vi "ToTable Test.vi"() -> (2 "Pass":bool)   [LabVIEW 2013, in "Table Manager tests.lvlib"]
uses:
  Table Manager tests.lvlib
  <vilib>/NI/Tag Bus/tag/Data Type.ctl
  editor node/Permissions Enum.ctl
  Listbox/Multi Column Listbox.lvclass
  Listbox/Multi Column Listbox.lvclass/Multi Column Listbox.ctl
  Table Manager/Table Manager.lvclass/Table Manager.ctl
  editor node/tag bus configurable plugin editor node.lvclass
  Listbox/Write Listbox.vi
  Table Manager/Write Top VI.vi
  <vilib>/NI/Tag Bus/tag/tag descriptor.lvclass
panel:
  out "error":errorcluster
  in  "Permissions":T1
  in  "data type":T2
  in  "Table":i32(listbox)
  out "error out":errorcluster
  out "table":string[][](array[string])
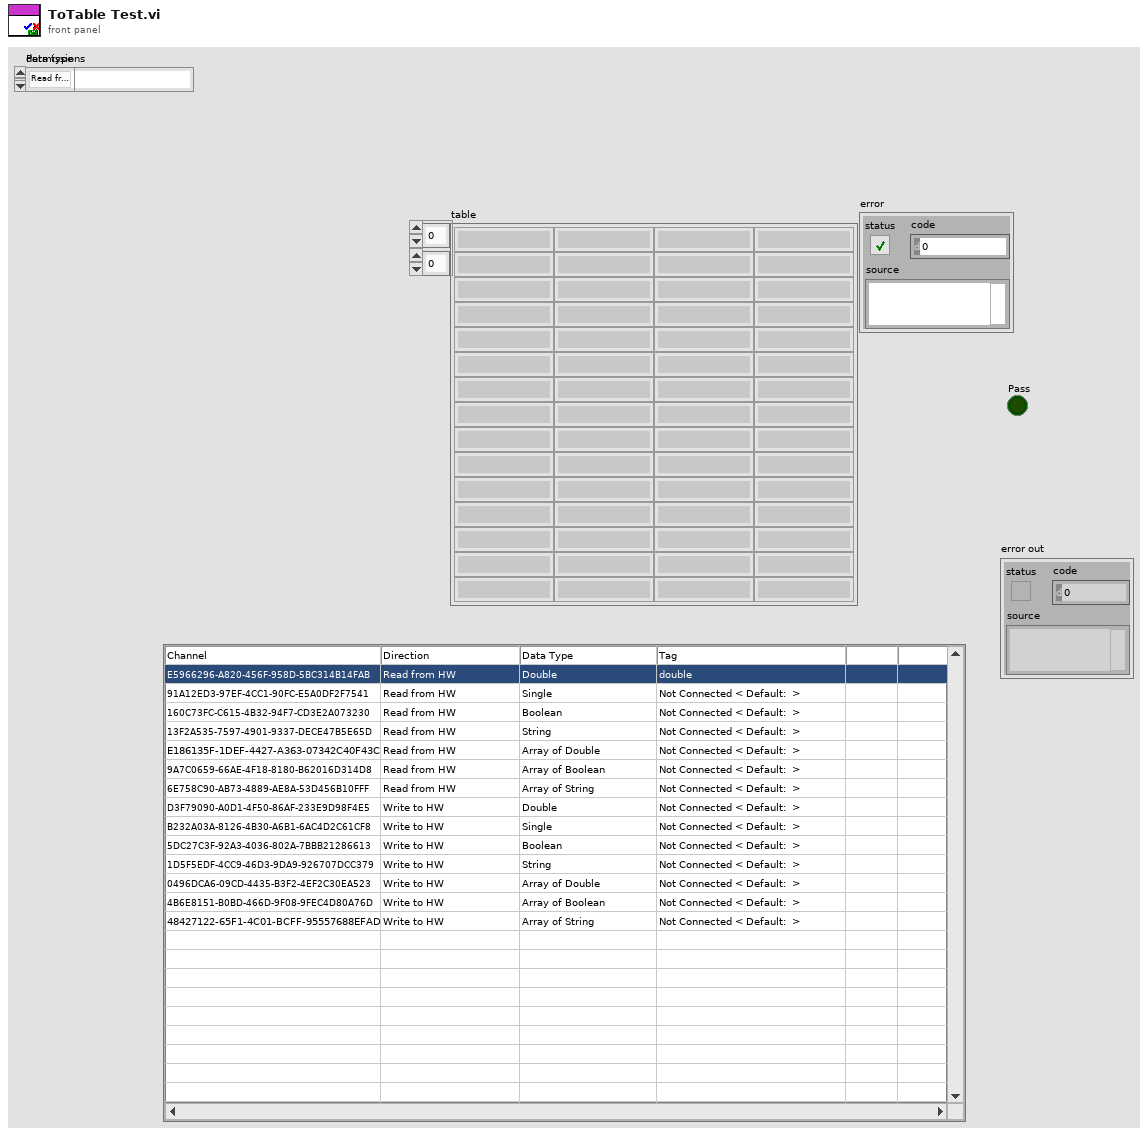
[diagram p1: front panel]
types:
  T1 = typedef "tag bus configurable plugin editor node.lvclass/Permissions Enum.ctl" = enum16{"Read from HW", "Write to HW"}
  T2 = typedef "tag bus.lvlib/tag descriptor.lvclass/Data Type.ctl" = enum16{"Double", "Single", "I64", "I32", "I16", "I8", "U64", "U32", "U16", "U8", "Boolean", "String", "Array of Double", "Array of Single", "Array of I64", "Array of I32", "Array of I16", "Array of I8", "Array of U64", "Array of U32", "Array of U16", "Array of U8", "Array of Boolean", "Array of String"}
  T3 = typedef "Table Manager.lvlib/Column.lvclass/Column Descriptor.ctl" = cluster{"name":string, "caption":string, "Column Type":T4, "Params":string, "AutoSizeMode":i32, "FillWeight":sgl, "MinWidth":u32, "tooltip":string, "Enum Reference":refnum<vi>, "Channel suffix":string, "Read Only":bool, "Call Back VI":T5, "DT Dependency":i32, "name dependency":i32, "data type":T2, "Custom Column":refnum<class "Column.lvclass">}
  T4 = typedef "Table Manager.lvlib/Column.lvclass/Column Type.ctl" = enum16{"String", "Mapping", "Enum", "Custom"}
  T5 = typedef "Table Manager.lvlib/Table Manager.lvclass/Call Back Ref Type Def.ctl" = refnum<vi>
  T6 = typedef "Table Manager.lvlib/Table Manager.lvclass/object ref.ctl" = cluster{"engine":refnum<data-value>, "Node Ref":refnum<data-value>}
  T7 = typedef "Table Manager.lvlib/Table Manager.lvclass/references.ctl" = cluster{"stop event":T8, "refresh UI":T9, "cache state":T10, "node change":T11, "user event out":refnum<user-event>, "main queue":T12, "user event":T13}
  T8 = typedef "NISE_CEF_Node.lvclass/StopEvent.ctl" = refnum<user-event>
  T9 = typedef "NISE_CEF_Node.lvclass/RefreshUIEvent.ctl" = refnum<user-event>
  T10 = typedef "NISE_CEF_Node.lvclass/CacheState.ctl" = refnum<user-event>
  T11 = typedef "NISE_CEF_Node.lvclass/NodeChangeEvent.ctl" = refnum<user-event>
  T12 = typedef "AMC.lvlib/Message Queue.ctl" = refnum<queue>
  T13 = typedef "NISE_CEF_Node.lvclass/UserEventRef.ctl" = refnum<user-event>
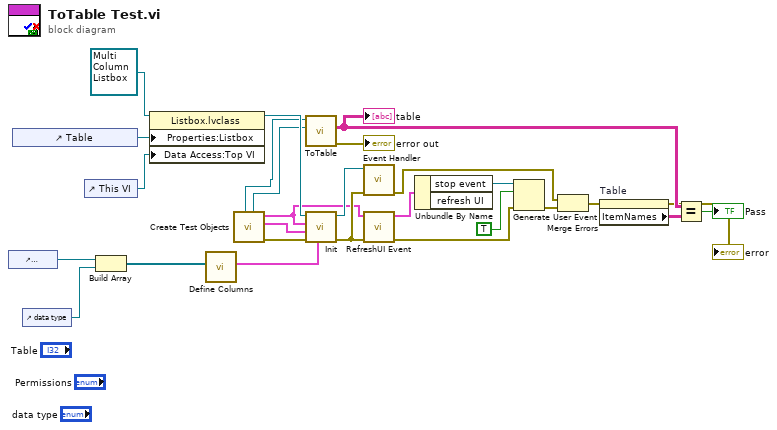
[diagram p0: block diagram]
diagram:
  n1 = control-ref of="Permissions"() -> (w21:refnum<vi>)
  n2 = control-ref of="Table"() -> (w25:refnum<vi>)
  n3 = control-ref of="data type"() -> (w20:refnum<vi>)
  n4 = control-ref of="This VI"() -> (w24:refnum<vi>)
  n5 = Build Array(w21, w20) -> (w19:refnum<vi>[])
  n6 = property class="Listbox.lvclass"(reference=refnum<class "Multi Column Listbox.lvclass"> refnum ("Table Manager.lvlib:Multi Column Listbox.lvclass"), "Properties:Listbox"=w25, "Data Access:Top VI"=w24) -> (reference out=w16:refnum<class "Multi Column Listbox.lvclass">)  [unwired: 1 in, 1 out]
  n7 = call "Define Columns.vi"("Enum Array"=w19) -> ("Column Definition"=w18:T3[])  [unwired: 10 in]
  n8 = call "Create Test Objects.vi"() -> ("error out"=w17:errorcluster, "Objects"=w3:T6, "Refs"=w4:T7, "engine configuration out"=w5:refnum<class "engine configuration.lvclass">, "tag bus configurable plugin editor node out"=w2:refnum<class "tag bus configurable plugin editor node.lvclass">)  [unwired: 7 in]
  n9 = call-dynamic "ToTable.vi"("variant"=w5, "node in"=w2) -> ("error out"=→"error out":errorcluster, "table"=w22:string[][])  [unwired: 6 in, 2 out]
  "table" <- w22
  n10 = call-dynamic "Init.vi"("Column Descriptors"=w18, "error in (no error)"=w17, "Node object refs"=w3, "Event References"=w4, "Multi Column Listbox in"=w16) -> ("error out"=w14:errorcluster, "Multi Column Listbox out"=w15:refnum<class "Multi Column Listbox.lvclass">)  [unwired: 4 in, 1 out]
  n11 = call-dynamic "Event Handler.vi"("error in"=w14, "Listbox in"=w15) -> ("error out"=w9:errorcluster)  [unwired: 8 in, 1 out]
  n12 = call "RefreshUI Event.vi"("error in (no error)"=w14, "References in"=w4) -> ("error out"=w11:errorcluster, "References out"=w13:T7)  [unwired: 8 in]
  n13 = Unbundle By Name(w13) -> ("stop event"=w12:T8)  [unwired: 1 out]
  n14 = Generate User Event(user event=w12, event data cluster=TRUE ("event data"), error in=w11) -> (error out=w10:errorcluster)  [unwired: 1 in, 1 out]
  n15 = Merge Errors(w9, w10) -> (w8:errorcluster)
  n16 = property on="Table" class="MCListbox (strict)"(error in=w8) -> (error out=→"error":errorcluster, "ItemNames"=w23:string[][])  [unwired: 1 in, 1 out]
  n17 = Equal?(x=w22, y=w23) -> (x = y?=→"Pass":bool)
